vi "Pcre2PatternInfoData8.vi"(8 "error in":errorcluster, 9 "size":i32, 10 "What":u32 format="%.0x", 11 "pCode":u64 format="%.0x") -> (0 "error out":errorcluster, 2 "DataBytes":u8[](array[numeric]) format="%02x", 3 "pCode":u64 format="%.0x")   [LabVIEW 2021, in "libpcre2-8.lvlib"]
uses:
  libpcre2-8.lvlib
  libpcre2-8-x32.dll
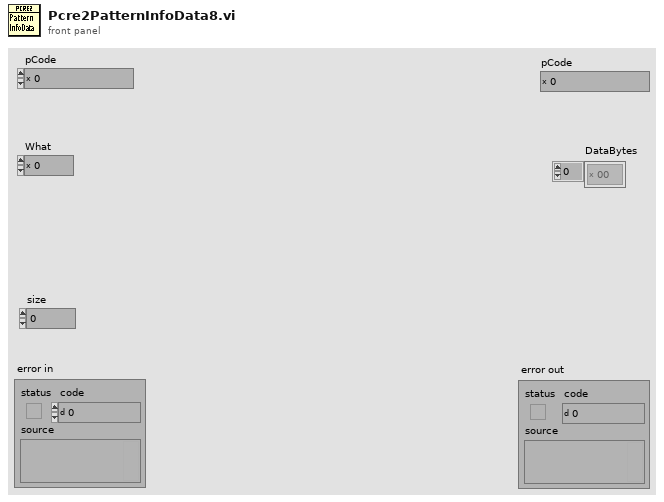
[diagram p1: front panel]
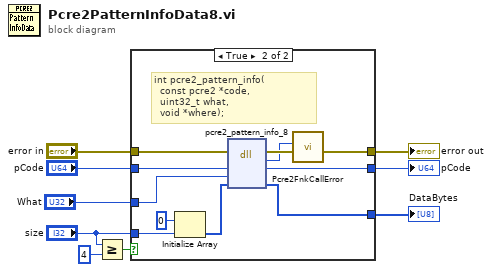
[diagram p0: block diagram]
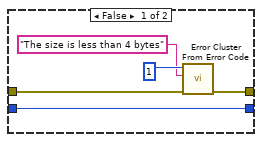
[diagram p2: hidden frame]
diagram:
  n1 = Greater Or Equal?(x="size", y=4) -> (x >= y?=w2:bool)
  n2 = case shown="True" w2 {
    tunnel: "error in" -> [w13 w25]
    tunnel: "pCode" -> [w12 w24]
    tunnel: [w12 w23] -> w8
    tunnel: "What" -> [_ w22]
    tunnel: [_ w20] -> w6
    tunnel: [w14 w18] -> w5
    tunnel: "size" -> [_ w16]
    frame False {
      n3 = call <vilib>:"Error Cluster From Error Code.vi"("error in (no error)"=w13, "error message (\"\")"="The size is less than 4 bytes" ("possible reason"), "error code (0)"=1 ("code (0)")) -> ("error out"=w14:errorcluster)  [unwired: 6 in]
    }
    frame True {
      # "int pcre2_pattern_info(\n  const pcre2 *code,\n  uint32_t what,\n  void *where);"
      n4 = Initialize Array(u8 0 ("U8"), w16) -> (w21:u8[])
      n5 = dll-call lib="libpcre2-8-x*.dll" fn="pcre2_pattern_info_8"(error in=w25, "code"=w24, "what"=w22, "where"=w21) -> (error out=w19:errorcluster, "return type"=w17:i32, "code"=w23:u64, "where"=w20:u8[])  [unwired: 3 in, 1 out]
      n6 = call "Pcre2FnkCallError.vi"("error in"=w19, "ErrorCode"=w17) -> ("error out"=w18:errorcluster)  [unwired: 9 in]
    }
  }
  "pCode" <- w8
  "error out" <- w5
  "DataBytes" <- w6
